vi "ROI entry-Obtain number of Z planes.vi"(8 "error in (no error)":errorcluster, 10 "Message string":string, 11 "Z-stack images folder path":path) -> (0 "error out":errorcluster, 2 "Number of planes":i32, 3 "Some planes found / Proceed":bool)   [LabVIEW 2017]
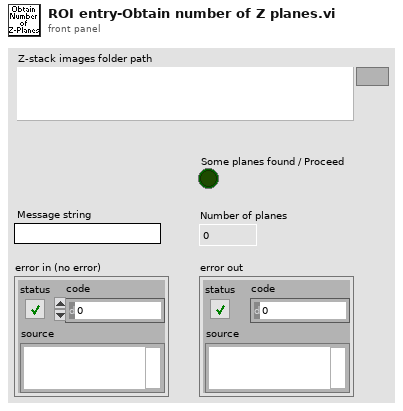
[diagram p1: front panel]
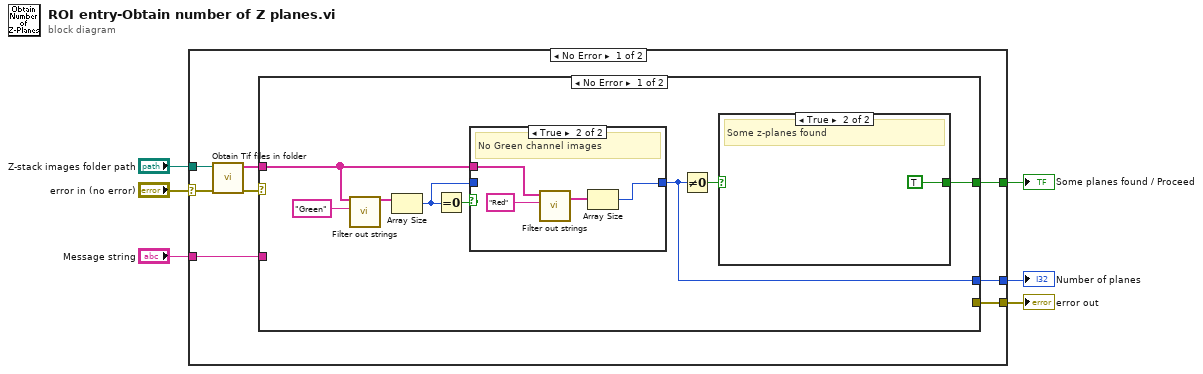
[diagram p0: block diagram]
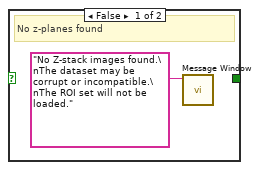
[diagram p2: hidden frame]
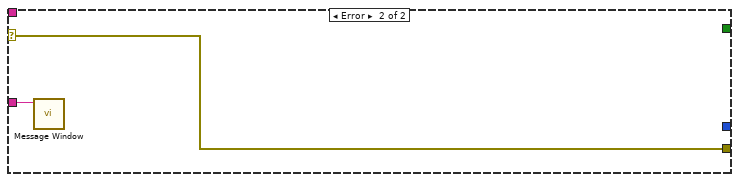
[diagram p4: hidden frame]
diagram:
  n1 = case shown="No Error" "error in (no error)" {
    selector: "error in (no error)" -> [w8 w32]
    tunnel: [w14 _] -> w6
    tunnel: "Message string" -> [w13 _]
    tunnel: [w12 w32] -> w4
    tunnel: "Z-stack images folder path" -> [w9 _]
    tunnel: [w7 _] -> w1
    frame No Error {
      n2 = call "Obtain Tif files in folder.vi"("error in"=w8, "Z-stack images folder path"=w9) -> ("error IO"=w11:errorcluster, "filenames (no extension)"=w10:string[])  [unwired: 7 in, 1 out]
      n3 = case shown="No Error" w11 {
        selector: w11 -> [_ w31]
        tunnel: w10 -> [w19 _]
        tunnel: [_ w31] -> w12
        tunnel: w13 -> [_ w30]
        tunnel: [w16 _] -> w14
        tunnel: [w15 _] -> w7
        frame No Error {
          n4 = call "Filter out strings.vi"("Filter out if containing this string"="Green", "array w/ subset deleted in"=w19) -> ("array w/ subset deleted out"=w21:string[])  [unwired: 9 in]
          n5 = Array Size(array=w21) -> (size(s)=w18:i32)
          n6 = Equal To 0?(x=w18) -> (x = 0?=w20:bool)
          n7 = case shown="True" w20 {
            tunnel: w19 -> [_ w27]
            tunnel: w18 -> [w25 _]
            tunnel: [w25 w26] -> w16
            frame False {
              # "Green channel images found"
            }
            frame True {
              # "No Green channel images"
              n8 = call "Filter out strings.vi"("Filter out if containing this string"="Red", "array w/ subset deleted in"=w27) -> ("array w/ subset deleted out"=w28:string[])  [unwired: 9 in]
              n9 = Array Size(array=w28) -> (size(s)=w26:i32)
            }
          }
          n10 = Not Equal To 0?(x=w16) -> (x != 0?=w17:bool)
          n11 = case shown="True" w17 {
            tunnel: [_ TRUE] -> w15
            frame False {
              # "No z-planes found"
              n12 = call "Message Window.vi"("Message string"="No Z-stack images found.\nThe dataset may be corrupt or incompatible.\nThe ROI set will not be loaded.") -> ()  [unwired: 10 in, 1 out]
            }
            frame True {
              # "Some z-planes found"
            }
          }
        }
        frame Error {
          n13 = call "Message Window.vi"("Message string"=w30) -> ()  [unwired: 10 in, 1 out]
        }
      }
    }
    frame Error {
    }
  }
  "Number of planes" <- w6
  "error out" <- w4
  "Some planes found / Proceed" <- w1
